vi "Kill UTP TEF.vi"() -> ()   [LabVIEW 2025]
panel:
  out "error out":errorcluster
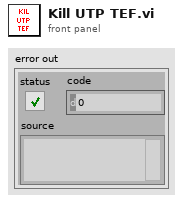
[diagram p1: front panel]
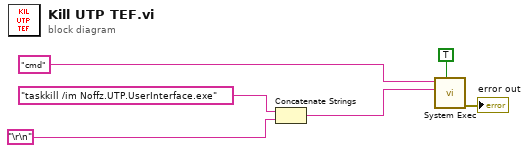
[diagram p0: block diagram]
diagram:
  n1 = Concatenate Strings("taskkill /im Noffz.UTP.UserInterface.exe" ("standard input"), "\r\n") -> (w1:string)
  n2 = call <vilib>:"System Exec.vi"("wait until completion? (T)"=TRUE, "standard input"=w1, "command line"="cmd") -> ("error out"=→"error out":errorcluster)  [unwired: 5 in, 3 out]
